vi "CPP_ReflectSingleSided.vi"(1 "SingleSidedData":dbl[](array[numeric])) -> (0 "ReflectedData":dbl[](array[numeric]))   [LabVIEW 2011]
doc: "Reflects single-sided spectral data for use with double-ended (Unshifted) FFTs. Duplicates the last point of the input sequence to ensure correct length."
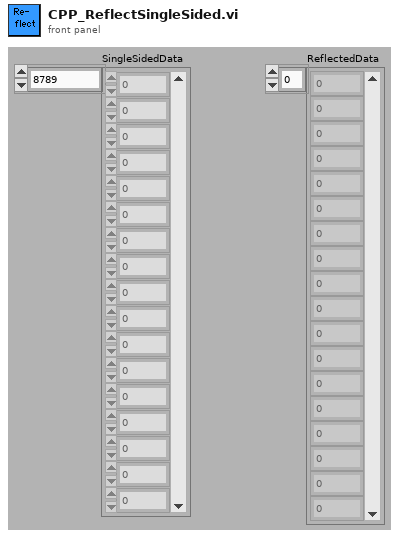
[diagram p1: front panel]
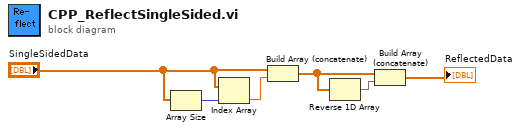
[diagram p0: block diagram]
diagram:
  n1 = Array Size(array="SingleSidedData") -> (size(s)=w3:i32)
  n2 = Index Array(array="SingleSidedData", index=w3) -> (element=w5:dbl)
  n3 = Build Array (concatenate)("SingleSidedData", w5) -> (w6:dbl[])
  n4 = Reverse 1D Array(array=w6) -> (reversed array=w1:dbl[])
  n5 = Build Array (concatenate)(w6, w1) -> (→"ReflectedData":dbl[])
